vi "Base64 To Base64-URL.vi"(11 "Base64 String":string) -> (3 "Base64-URL String":string)   [LabVIEW 2020, in "Base64.lvlib"]
uses:
  Base64.lvlib
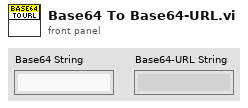
[diagram p1: front panel]
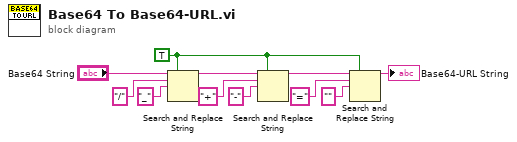
[diagram p0: block diagram]
diagram:
  w2 = TRUE ("replace all? (F)")
  n1 = Search and Replace String(replace all?=w2, input string="Base64 String", search string="/", replace string="_" ("search string")) -> (result string=w4:string)  [unwired: 4 in, 3 out]
  n2 = Search and Replace String(replace all?=w2, input string=w4, search string="+", replace string="-" ("search string")) -> (result string=w3:string)  [unwired: 4 in, 3 out]
  n3 = Search and Replace String(replace all?=w2, input string=w3, search string="=", replace string="" ("search string")) -> (result string=→"Base64-URL String":string)  [unwired: 4 in, 3 out]
